vi "Main On Compile Action VI.vi"(8 "error in (no error)":errorcluster, 11 "Device Item Ref in":T1 format="%.0x") -> (0 "error out":errorcluster)   [LabVIEW 2016, in "Ballard Arinc-429 System Explorer.lvlib"]
uses:
  Ballard Arinc-429 System Explorer.lvlib
  <vilib>/WebDAVClient/NI_WebDAV.lvlib
  <vilib>/WebDAVClient/Advanced/FileInfo.ctl
  <vilib>/NI Veristand/Custom Device API/Custom Device API.lvlib
  <vilib>/NI Veristand/Custom Device API/Get Item Property (I32).vi
  Shared/Controls and Global/Global.vi
  Shared/Ballard Arinc-429 Shared.lvlib
  <vilib>/NI Veristand/Custom Device API/Set Item Property (Variant).vi
  <vilib>/NI Veristand/Custom Device API/Custom Device Channel Type.ctl
  <vilib>/NI Veristand/Custom Device API/Custom Device Item Ref.ctl
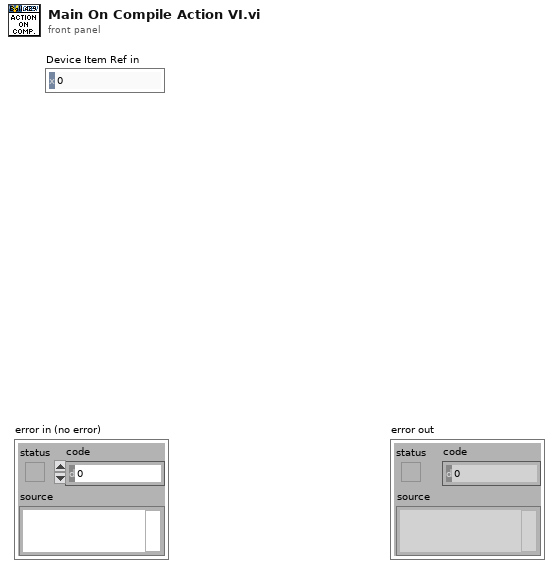
[diagram p1: front panel]
types:
  T1 = typedef "Custom Device API.lvlib/Custom Device Item Ref.ctl" = u64
  T2 = typedef "NI_WebDAV.lvlib/FileInfo.ctl" = cluster{"type":string, "size":u64, "last modification":timestamp, "display name":string, "uri":string}
  T3 = typedef "Custom Device API.lvlib/Custom Device Channel Type.ctl" = enum16{"Input", "Output"}
  T4 = typedef "NI_WebDAV.lvlib/SessionHandle.ctl" = refnum<k1>
  T5 = typedef "Ballard Arinc-429 Engine.lvlib/RT HW Channel.ctl" = cluster{"Labels Settings":T6[], "channel handle":u32, "channel #":u16}
  T6 = typedef "Ballard Arinc-429 Engine.lvlib/RT Label Settings.ctl" = cluster{"Name":string, "xmlName":string, "Label":T7, "transferPeriod":T8, "SDI_Enabled":bool, "SDI":u8, "Word":T9, "TransferType":T13, "has timestamp?":bool, "LBL Disable Index":i32, "Message Handle":u64, "Initialized?":bool, "Word Initial Raw Value":u32}
  T7 = typedef "Ballard Arinc-429 Shared.lvlib/Label.ctl" = u8
  T8 = typedef "Ballard Arinc-429 Shared.lvlib/transferPeriod.ctl" = u32
  T9 = typedef "Ballard Arinc-429 Engine.lvlib/RT Word Settings.ctl" = cluster{"Param Setting":T10}
  T10 = typedef "Ballard Arinc-429 Engine.lvlib/RT Param Setting.ctl" = cluster{"Start Bit":T11[], "Num Bits":T12[], "Signed?":bool[], "ScaleFac":dbl[], "ScaleOffset":dbl[], "Channel FIFO Buffer Index":i32[], "Encoding":enum16{"BNR", "BCD", "Discrete"}[]}
  T11 = typedef "Ballard Arinc-429 Shared.lvlib/Start Bit.ctl" = i32
  T12 = typedef "Ballard Arinc-429 Shared.lvlib/Number of Bits.ctl" = i32
  T13 = typedef "Ballard Arinc-429 Shared.lvlib/TransferType.ctl" = enum16{"ScheduledLabel", "Acyclic", "Block", "Strobe"}
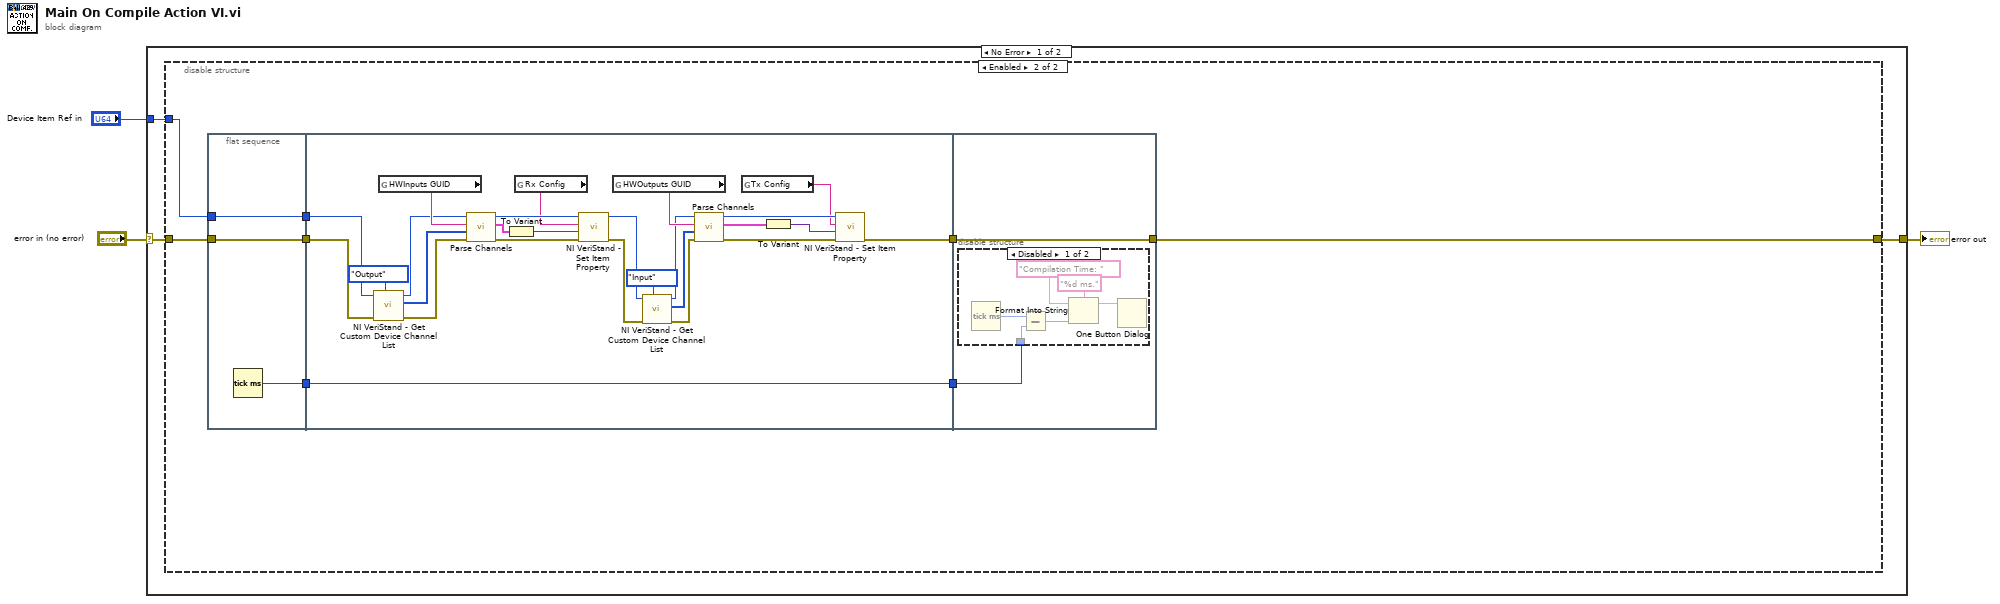
[diagram p0: block diagram]
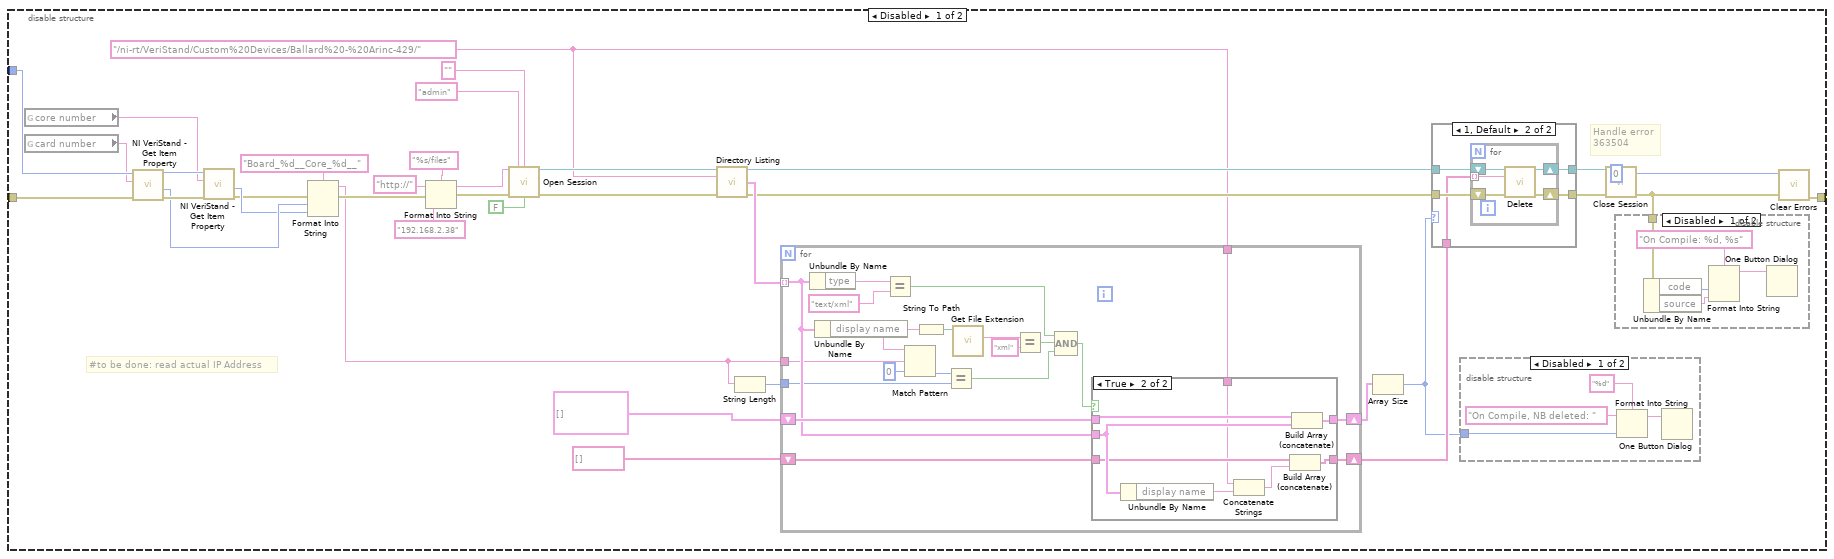
[diagram p2: hidden frame]
diagram:
  n1 = case shown="No Error" "error in (no error)" {
    selector: "error in (no error)" -> [w6 w140]
    tunnel: [w4 w140] -> w3
    tunnel: "Device Item Ref in" -> [w5 _]
    frame No Error {
      n2 = disable-structure shown="Enabled" {
        disable-tunnel: w6 -> [w43 w101]
        disable-tunnel: w5 -> [w41 w102]
        disable-tunnel: [w18 w100] -> w4
        frame Disabled {
          w7 = "/ni-rt/VeriStand/Custom%20Devices/Ballard%20-%20Arinc-429/" ("Remote Data Folder")
          # "#to be done: read actual IP Address"
          # "Handle error\n363504"
          n3 = global read "Global.vi" "core number"() -> (w38:string)
          n4 = global read "Global.vi" "card number"() -> (w39:string)
          n5 = call-poly <vilib>:"NI VeriStand - Get Item Property.vi"("error in (no error)"=w43, "Property Name"=w39, "Item Ref in"=w41) -> ("error out"=w42:errorcluster, "Value"=w36:i32, "Item Ref out"=w40:T1)  [unwired: 5 in, 1 out]
          n6 = call-poly <vilib>:"NI VeriStand - Get Item Property.vi"("error in (no error)"=w42, "Property Name"=w38, "Item Ref in"=w40) -> ("error out"=w34:errorcluster, "Value"=w35:i32)  [unwired: 5 in, 2 out]
          n7 = Format Into String(format string="Board_%d__Core_%d__", error in=w34, w36, w35) -> (resulting string=w20:string, error out=w26:errorcluster)  [unwired: 1 in]
          n8 = Format Into String(format string="%s/files" ("Host Address"), initial string="http://" ("Host Address"), error in=w26, "192.168.2.38" ("Host Address")) -> (resulting string=w24:string, error out=w23:errorcluster)
          n9 = call <vilib>:"Open Session.vi"("host uri prefix"=w24, "username"="admin" ("Username"), "password"="" ("Password"), "error in (no error)"=w23, "verify server?"=FALSE) -> ("session handle out"=w30:T4, "error out"=w29:errorcluster)  [unwired: 9 in]
          n10 = call <vilib>:"Directory Listing.vi"("session handle"=w30, "relative uri"=w7, "error in (no error)"=w29) -> ("session handle out"=w13:T4, "file list"=w28:T2[], "error out"=w15:errorcluster)  [unwired: 9 in, 1 out]
          n11 = String Length(string=w20) -> (length=w19:i32)
          n12 = for {
            tunnel: w28 -> [w74] mode=indexing
            shift-right: [w79] -> w16
            shift-left: T2[] [] ("file list") -> [w75]
            tunnel: w20 -> [w72]
            tunnel: w19 -> [w69]
            shift-right: [w66] -> w10
            shift-left: string[] [] -> [w67]
            tunnel: w7 -> [w65]
            n13 = Unbundle By Name(w74) -> ("type"=w84:string)
            n14 = Unbundle By Name(w74) -> ("display name"=w73:string)
            n15 = Equal?(x=w84, y="text/xml") -> (x = y?=w77:bool)
            n16 = Match Pattern(string=w73, regular expression=w72, offset (0)=0) -> (offset past match=w70:i32)  [unwired: 3 out]
            n17 = String To Path(string=w73) -> (path=w82:path)
            n18 = Equal?(x=w70, y=w69) -> (x = y?=w68:bool)
            n19 = call <vilib>:"Get File Extension.vi"("file"=w82) -> ("lowercase file extension"=w81:string)  [unwired: 6 in, 4 out]
            n20 = Equal?(x=w81, y="xml") -> (x = y?=w78:bool)
            n21 = Compound Arithmetic op=AND(w77, w78, w68) -> (w76:bool)
            n22 = case shown="True" w76 {
              tunnel: [w86 w94] -> w79
              tunnel: w75 -> [w86 w93]
              tunnel: w74 -> [_ w92]
              tunnel: w67 -> [w85 w91]
              tunnel: [w85 w90] -> w66
              tunnel: w65 -> [_ w88]
              frame False {
              }
              frame True {
                n23 = Unbundle By Name(w92) -> ("display name"=w89:string)
                n24 = Concatenate Strings(w88, w89) -> (w87:string)
                n25 = Build Array (concatenate)(w91, w87) -> (w90:string[])
                n26 = Build Array (concatenate)(w93, w92) -> (w94:T2[])
              }
            }
          }
          n27 = Array Size(array=w16) -> (size(s)=w9:i32)
          n28 = case shown="1, Default" w9 {
            tunnel: w15 -> [w54 w58]
            tunnel: [w54 w57] -> w14
            tunnel: w13 -> [w53 w59]
            tunnel: [w53 w56] -> w12
            tunnel: w10 -> [_ w55]
            frame 0 {
            }
            frame 1, Default {
              n29 = for {
                tunnel: w55 -> [w60] mode=indexing
                shift-right: [w61] -> w56
                shift-left: w59 -> [w64]
                shift-right: [w62] -> w57
                shift-left: w58 -> [w63]
                n30 = call <vilib>:"Delete.vi"("session handle"=w64, "relative uri"=w60, "error in (no error)"=w63) -> ("session handle out"=w61:T4, "error out"=w62:errorcluster)  [unwired: 11 in]
              }
            }
          }
          n31 = disable-structure shown="Disabled" {
            disable-tunnel: w9 -> [w50 _]
            frame Disabled {
              n32 = Format Into String(format string="%d", initial string="On Compile, NB deleted: ", w50) -> (resulting string=w51:string)  [unwired: 1 in, 1 out]
              n33 = One Button Dialog(message=w51) -> ()  [unwired: 1 in, 1 out]
            }
            frame Enabled {
            }
          }
          n34 = call <vilib>:"Close Session.vi"("session handle"=w12, "error in (no error)"=w14) -> ("error out"=w8:errorcluster)  [unwired: 13 in]
          n35 = disable-structure shown="Disabled" {
            disable-tunnel: w8 -> [w48 _]
            frame Disabled {
              n36 = Unbundle By Name(w48) -> ("code"=w46:i32, "source"=w45:string)
              n37 = Format Into String(format string="On Compile: %d, %s", w46, w45) -> (resulting string=w44:string)  [unwired: 2 in, 1 out]
              n38 = One Button Dialog(message=w44) -> ()  [unwired: 1 in, 1 out]
            }
            frame Enabled {
            }
          }
          n39 = call <vilib>:"Clear Errors.vi"("error in (no error)"=w8, "specific error code to clear (0: all)"=0) -> ("error out"=w18:errorcluster)  [unwired: 4 in, 1 out]
        }
        frame Enabled {
          n40 = flat-sequence {
            tunnel: w101 -> [w104]
            tunnel: w102 -> [w105]
            tunnel: [w105] -> w99
            tunnel: [w104] -> w98
            tunnel: [w103] -> w96
            tunnel: w99 -> [w117]
            tunnel: w98 -> [w116]
            tunnel: [w122] -> w97
            tunnel: w96 -> [w118]
            tunnel: [w118] -> w95
            tunnel: [w133] -> w100
            tunnel: w97 -> [w133]
            tunnel: w95 -> [w132]
            frame #0 {
              n41 = Tick Count (ms)() -> (millisecond timer value=w103:u32)
            }
            frame #1 {
              n42 = call <vilib>:"NI VeriStand - Get Custom Device Channel List.vi"("Channel Type"=Custom_Device_Channel_Type."Output", "error in (no error)"=w116, "Device Ref in"=w117) -> ("error out"=w115:errorcluster, "Specified Channel Ref List"=w108:T1[], "Device Ref out"=w114:T1)  [unwired: 6 out]
              n43 = global read "Global.vi" "HWInputs GUID"() -> (w130:string)
              n44 = call "Parse Channels.vi"("error in (no error)"=w115, "Specified Channel Ref List"=w108, "Section GUID"=w130, "Device Reference in"=w114) -> ("error out"=w124:errorcluster, "Channel Data []"=w126:T5[], "Device Reference out"=w128:T1)  [unwired: 4 in, 1 out]
              n45 = To Variant(anything=w126) -> (Variant=w125:variant)
              n46 = global read "Global.vi" "Rx Config"() -> (w127:string)
              n47 = call-poly <vilib>:"NI VeriStand - Set Item Property.vi"("error in (no error)"=w124, "Value"=w125, "Property Name"=w127, "Item Ref in"=w128) -> ("error out"=w111:errorcluster, "Item Ref out"=w107:T1)  [unwired: 5 in, 1 out]
              n48 = global read "Global.vi" "HWOutputs GUID"() -> (w131:string)
              n49 = call <vilib>:"NI VeriStand - Get Custom Device Channel List.vi"("Channel Type"=Custom_Device_Channel_Type."Input", "error in (no error)"=w111, "Device Ref in"=w107) -> ("error out"=w110:errorcluster, "Specified Channel Ref List"=w109:T1[], "Device Ref out"=w106:T1)  [unwired: 6 out]
              n50 = call "Parse Channels.vi"("error in (no error)"=w110, "Specified Channel Ref List"=w109, "Section GUID"=w131, "Device Reference in"=w106) -> ("error out"=w123:errorcluster, "Channel Data []"=w120:T5[], "Device Reference out"=w129:T1)  [unwired: 4 in, 1 out]
              n51 = global read "Global.vi" "Tx Config"() -> (w121:string)
              n52 = To Variant(anything=w120) -> (Variant=w119:variant)
              n53 = call-poly <vilib>:"NI VeriStand - Set Item Property.vi"("error in (no error)"=w123, "Value"=w119, "Property Name"=w121, "Item Ref in"=w129) -> ("error out"=w122:errorcluster)  [unwired: 5 in, 2 out]
            }
            frame #2 {
              n54 = disable-structure shown="Disabled" {
                disable-tunnel: w132 -> [w138 _]
                frame Disabled {
                  n55 = Tick Count (ms)() -> (millisecond timer value=w139:u32)
                  n56 = Subtract(x=w139, y=w138) -> (x-y=w137:u32)
                  n57 = Format Into String(format string="%d ms.", initial string="Compilation Time: ", w137) -> (resulting string=w136:string)  [unwired: 1 in, 1 out]
                  n58 = One Button Dialog(message=w136) -> ()  [unwired: 1 in, 1 out]
                }
                frame Enabled {
                }
              }
            }
          }
        }
      }
    }
    frame Error {
    }
  }
  "error out" <- w3
